vi "getItem.vi"(8 "error in (no error)":errorcluster, 10 "Key":string, 11 "Bucket in":refnum<class "Bucket.lvclass">) -> (0 "error out":errorcluster, 2 "Value":variant, 3 "Bucket out":refnum<class "Bucket.lvclass">)   [LabVIEW 2017, in "Bucket.lvclass"]
uses:
  <userlib>/836-Library/Data_Structures/HashMap/Support/Bucket/Bucket.lvclass
  <userlib>/836-Library/Data_Structures/HashMap/Support/Bucket/Bucket.lvclass/Bucket.ctl
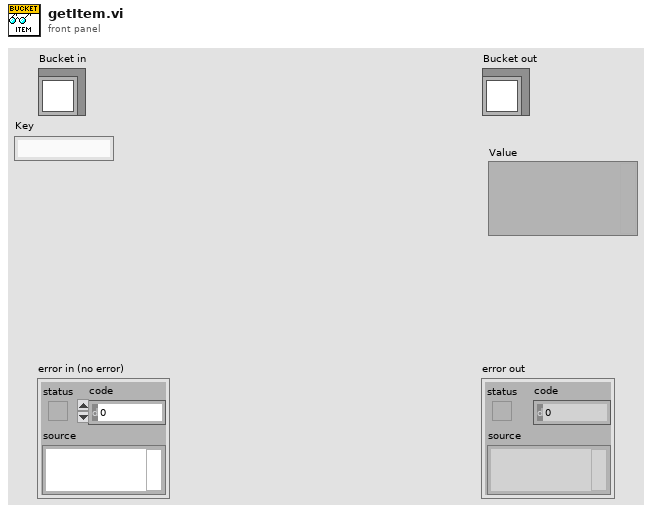
[diagram p1: front panel]
types:
  T1 = typedef "KeyValuePair.ctl" = cluster{"Key":string, "Value":variant}
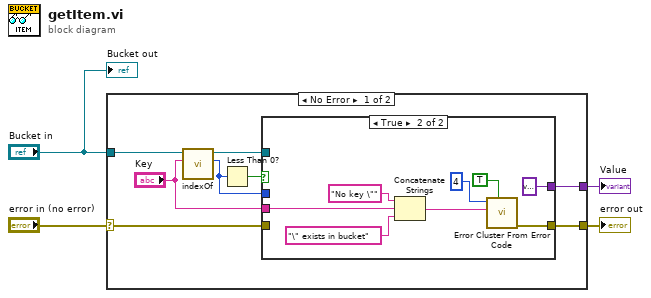
[diagram p0: block diagram]
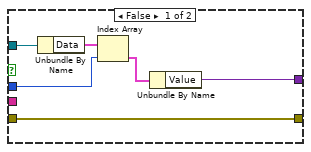
[diagram p2: hidden frame]
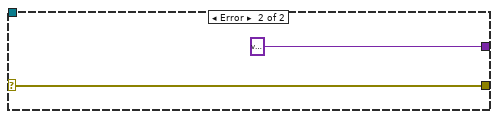
[diagram p3: hidden frame]
diagram:
  n1 = case shown="No Error" "error in (no error)" {
    selector: "error in (no error)" -> [w6 w28]
    tunnel: [w7 w28] -> w3
    tunnel: "Bucket in" -> [w12 _]
    tunnel: [w8 variant ("Value")] -> w2
    frame No Error {
      n2 = call <userlib>:"indexOf.vi"("Key"="Key", "Bucket in"=w12) -> ("Index"=w9:i32, "Bucket out"=w10:refnum<class "Bucket.lvclass">)  [unwired: 7 in, 1 out]
      n3 = Less Than 0?(x=w9) -> (x < 0?=w11:bool)
      n4 = case shown="True" w11 {
        tunnel: w10 -> [w18 _]
        tunnel: w9 -> [w16 _]
        tunnel: [w14 variant ("Value")] -> w8
        tunnel: [w13 w25] -> w7
        tunnel: w6 -> [w13 _]
        tunnel: "Key" -> [_ w21]
        frame False {
          n5 = Unbundle By Name(w18) -> ("Data"=w17:T1[])
          n6 = Index Array(array=w17, index=w16) -> (element=w15:T1)
          n7 = Unbundle By Name(w15) -> ("Value"=w14:variant)
        }
        frame True {
          n8 = Concatenate Strings("No key \"" ("string"), w21, "\" exists in bucket" ("string")) -> (w22:string)
          n9 = call <vilib>:"Error Cluster From Error Code.vi"("show call chain? (False)"=TRUE, "error message (\"\")"=w22, "error code (0)"=4) -> ("error out"=w25:errorcluster)  [unwired: 6 in]
        }
      }
    }
    frame Error {
    }
  }
  "error out" <- w3
  "Value" <- w2
  "Bucket out" <- "Bucket in"
